vi "Tx_Create FIFO Association - Acyclic Labels - Parameters Channels.vi"(8 "error in (no error)":errorcluster, 11 "Input Channel Data []":T5[](array[typedef]) {"Labels Settings"."Label Timestamp Channel Data Reference" format="%.0x"; "Labels Settings"."Label Disable/Trigger Channel Reference" format="%.0x"; "Labels Settings"."Word"."Param Setting"."Item Refs" format="%.0x"; "Labels Settings"."Word"."Param Setting"."Num Bits" min=1 max=32; "Labels Settings"."Word"."Param Setting"."Start Bit" min=8 max=31; "Labels Settings"."Label" format="%.0o"}) -> (0 "error out":errorcluster, 2 "Raw Values":T1, 3 "Map":T4[](array[typedef]) {"Channel Data Reference" format="%.0x"})   [LabVIEW 2020, in "Ballard Arinc-429 Engine.lvlib"]
doc: "This VI creates a static association between NI-VS FIFO Channel Index and Physical Channel, Label Index, Parameter Index for an Acyclic Tx Label."
uses:
  Ballard Arinc-429 Engine.lvlib
  Shared/Controls and Global/RT HW Channel.ctl
  Shared/Controls and Global/RT Label Settings.ctl
  Shared/Controls and Global/Label.ctl
  Shared/Controls and Global/transferPeriod.ctl
  Shared/Controls and Global/RT Word Settings.ctl
  Shared/Controls and Global/RT Param Setting.ctl
  Shared/Controls and Global/Start Bit.ctl
  Shared/Controls and Global/Number of Bits.ctl
  <vilib>/NI VeriStand/Custom Device API/Block Data Reference.ctl
  <vilib>/NI VeriStand/Custom Device API/Data Reference.ctl
  <vilib>/NI VeriStand/Custom Device API/Custom Device Item Ref.ctl
  Shared/Controls and Global/TransferType.ctl
  RT Controls/RT Tx Association.ctl
  RT Controls/RT Tx Default Raw Value.ctl
  RT Controls/RT Tx Default Raw Value_Association.ctl
  <vilib>/NI VeriStand/Custom Device API/Custom Device API.lvlib
  Shared/Ballard Arinc-429 Shared.lvlib
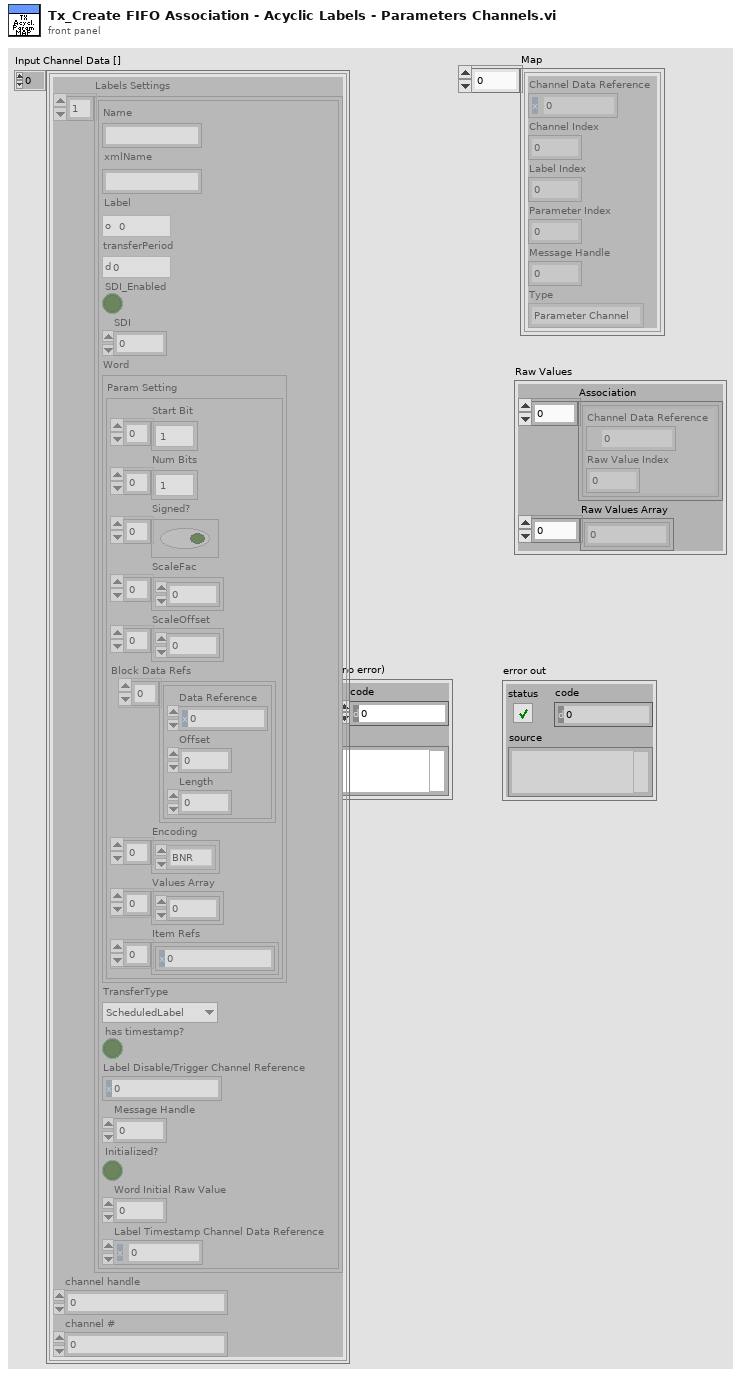
[diagram p1: front panel]
types:
  T1 = typedef "Ballard Arinc-429 Engine.lvlib/RT Tx Default Raw Value.ctl" = cluster{"Association":T2[], "Raw Values Array":u32[]}
  T2 = typedef "Ballard Arinc-429 Engine.lvlib/RT Tx Default Raw Value_Association.ctl" = cluster{"Channel Data Reference":T3, "Raw Value Index":i32}
  T3 = typedef "Custom Device API.lvlib/Data Reference.ctl" = i32
  T4 = typedef "Ballard Arinc-429 Engine.lvlib/RT Tx Association.ctl" = cluster{"Channel Data Reference":T3, "Channel Index":i32, "Label Index":i32, "Parameter Index":i32, "Message Handle":u64, "Type":enum16{"Parameter Channel", "Disable/Trigger Channel"}}
  T5 = typedef "Ballard Arinc-429 Shared.lvlib/RT HW Channel.ctl" = cluster{"Labels Settings":T6[], "channel handle":u64, "channel #":u16}
  T6 = typedef "Ballard Arinc-429 Shared.lvlib/RT Label Settings.ctl" = cluster{"Name":string, "xmlName":string, "Label":T7, "transferPeriod":T8, "SDI_Enabled":bool, "SDI":u8, "Word":T9, "TransferType":T15, "has timestamp?":bool, "Label Disable/Trigger Channel Reference":T14, "Message Handle":u64, "Initialized?":bool, "Word Initial Raw Value":u32, "Label Timestamp Channel Data Reference":T3}
  T7 = typedef "Ballard Arinc-429 Shared.lvlib/Label.ctl" = u8
  T8 = typedef "Ballard Arinc-429 Shared.lvlib/transferPeriod.ctl" = u32
  T9 = typedef "Ballard Arinc-429 Shared.lvlib/RT Word Settings.ctl" = cluster{"Param Setting":T10}
  T10 = typedef "Ballard Arinc-429 Shared.lvlib/RT Param Setting.ctl" = cluster{"Start Bit":T11[], "Num Bits":T12[], "Signed?":bool[], "ScaleFac":dbl[], "ScaleOffset":dbl[], "Block Data Refs":T13[], "Encoding":enum16{"BNR", "BCD", "Discrete"}[], "Values Array":dbl[], "Item Refs":T14[]}
  T11 = typedef "Ballard Arinc-429 Shared.lvlib/Start Bit.ctl" = i32
  T12 = typedef "Ballard Arinc-429 Shared.lvlib/Number of Bits.ctl" = i32
  T13 = typedef "Custom Device API.lvlib/Block Data Reference.ctl" = cluster{"Data Reference":T3, "Offset":u64, "Length":u64}
  T14 = typedef "Custom Device API.lvlib/Custom Device Item Ref.ctl" = u64
  T15 = typedef "Ballard Arinc-429 Shared.lvlib/TransferType.ctl" = enum16{"ScheduledLabel", "Acyclic", "Block", "Strobe"}
  T16 = enum16{"Parameter Channel", "Disable/Trigger Channel"}
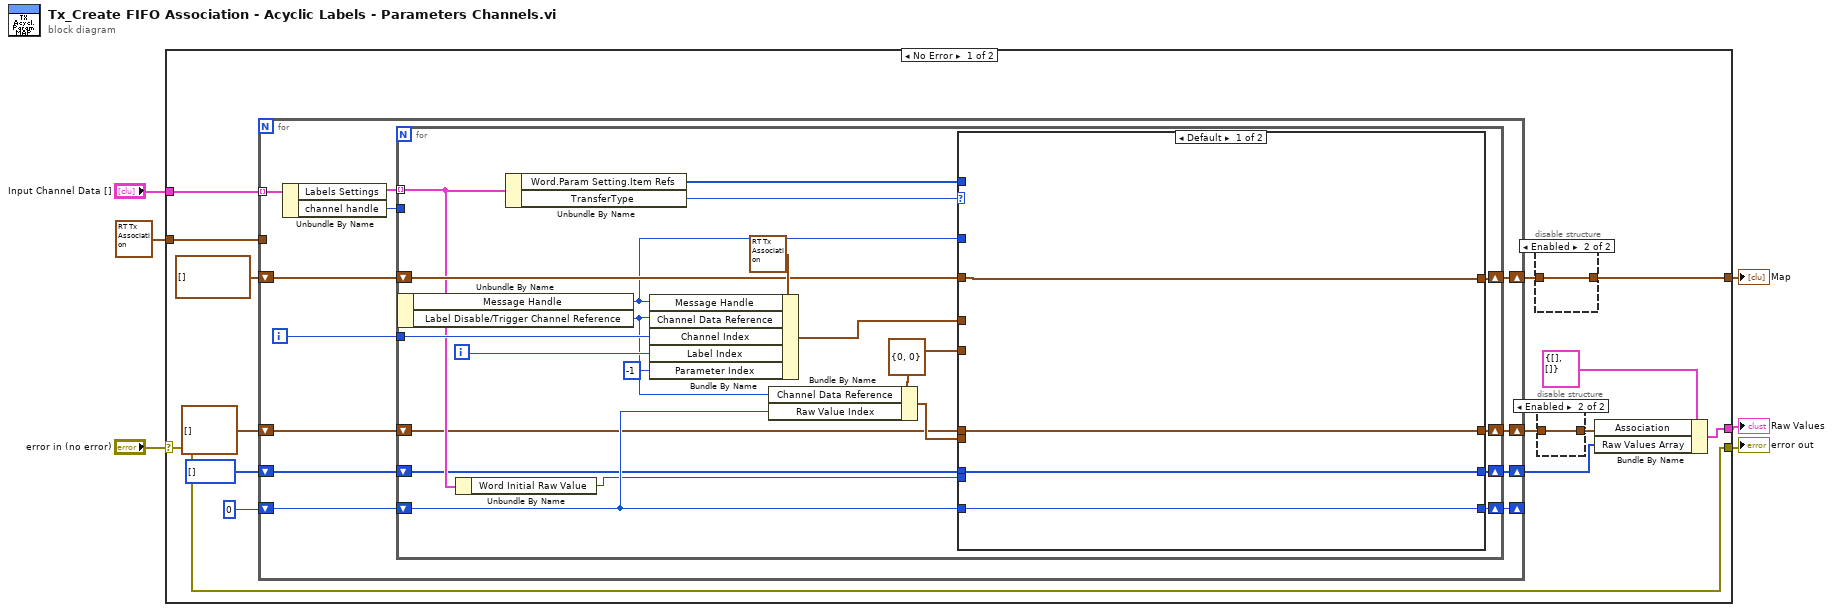
[diagram p0: block diagram]
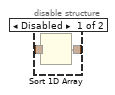
[diagram p2: hidden frame]
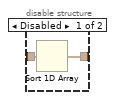
[diagram p3: hidden frame]
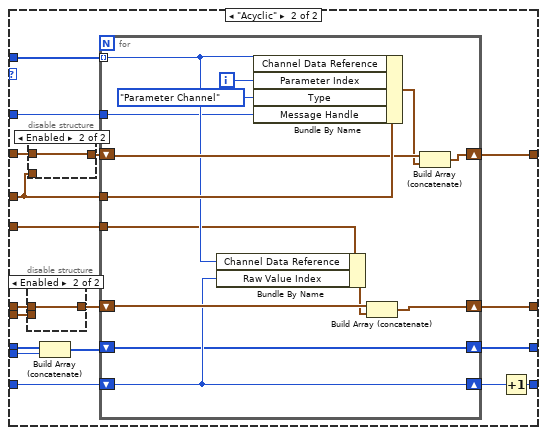
[diagram p4: hidden frame]
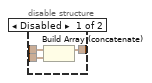
[diagram p5: hidden frame]
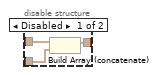
[diagram p6: hidden frame]
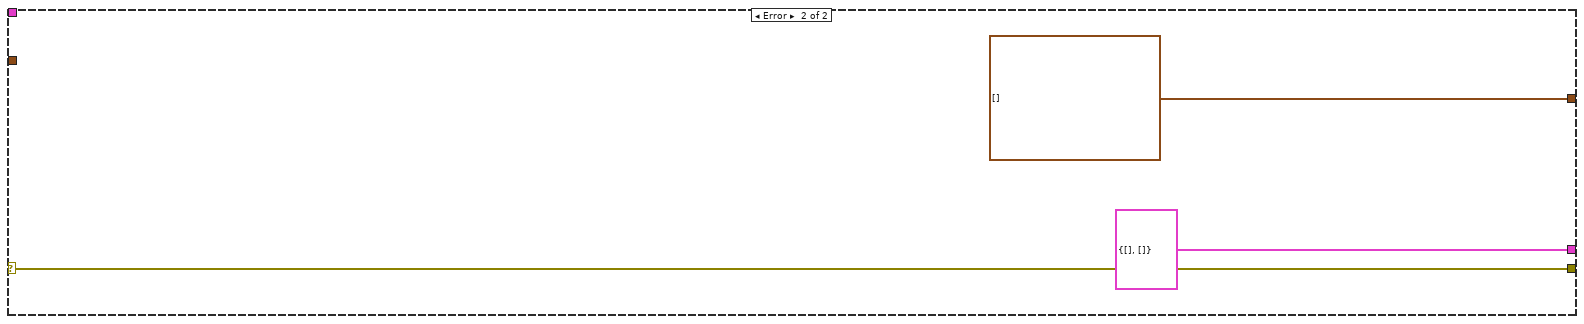
[diagram p7: hidden frame]
diagram:
  n1 = case shown="No Error" "error in (no error)" {
    selector: "error in (no error)" -> [w17 w106]
    tunnel: [w17 w106] -> w5
    tunnel: "Input Channel Data []" -> [w20 _]
    tunnel: T4 {"Channel Data Reference"=0, "Channel Index"=0, "Label Index"=0, "Parameter Index"=0, "Message Handle"=0, "Type"=enum."Parameter Channel"} ("Association") -> [w19 _]
    tunnel: [w16 T4[] []] -> w2
    tunnel: [w12 T1 {"Association"=[], "Raw Values Array"=[]}] -> w1
    frame No Error {
      n2 = for {
        tunnel: w20 -> [w37] mode=indexing
        tunnel: w19 -> [_]
        shift-right: [w34] -> w9
        shift-left: T4[] [] -> [w36]
        shift-right: [w32] -> w8
        shift-left: T2[] [] -> [w33]
        shift-right: [w28] -> w7
        shift-left: u32[] [] -> [w31]
        shift-right: [w29] -> _
        shift-left: 0 -> [w30]
        i -> [w35]
        n3 = Unbundle By Name(w37) -> ("Labels Settings"=w38:T6[], "channel handle"=w27:u64)
        n4 = for {
          tunnel: w38 -> [w51] mode=indexing
          shift-right: [w56] -> w34
          shift-left: w36 -> [w57]
          tunnel: w35 -> [w58]
          shift-right: [w52] -> w32
          shift-left: w33 -> [w45]
          shift-right: [w50] -> w28
          shift-left: w31 -> [w44]
          shift-right: [w49] -> w29
          shift-left: w30 -> [w48]
          tunnel: w27 -> [_]
          i -> [w53]
          w47 = T2 {"Channel Data Reference"=0, "Raw Value Index"=0}
          n5 = Unbundle By Name(w51) -> ("Message Handle"=w41:u64, "Label Disable/Trigger Channel Reference"=w42:T14)
          n6 = Unbundle By Name(w51) -> ("Word Initial Raw Value"=w43:u32)
          n7 = Unbundle By Name(w51) -> ("Word.Param Setting.Item Refs"=w54:T14[], "TransferType"=w40:T15)
          n8 = Bundle By Name(cluster=T4 {"Channel Data Reference"=0, "Channel Index"=0, "Label Index"=0, "Parameter Index"=-1, "Message Handle"=0, "Type"=enum."Disable/Trigger Channel"} ("Association"), "Message Handle"=w41, "Channel Data Reference"=w42, "Channel Index"=w58, "Label Index"=w53, "Parameter Index"=-1) -> (w55:T4)
          n9 = Bundle By Name(cluster=w47, "Channel Data Reference"=w42, "Raw Value Index"=w48) -> (w46:T2)
          n10 = case shown="Default" w40 {
            tunnel: w57 -> [w63 w81]
            tunnel: [w63 w79] -> w56
            tunnel: w55 -> [_ w78]
            tunnel: w54 -> [_ w77]
            tunnel: [w62 w76] -> w52
            tunnel: [w61 w75] -> w50
            tunnel: [w60 w73] -> w49
            tunnel: w48 -> [w60 w72]
            tunnel: w47 -> [_ w71]
            tunnel: w46 -> [_ w70]
            tunnel: w45 -> [w62 w69]
            tunnel: w44 -> [w61 w67]
            tunnel: w43 -> [_ w66]
            tunnel: w41 -> [_ w64]
            frame Default {
            }
            frame "Acyclic" {
              n11 = disable-structure shown="Enabled" {
                disable-tunnel: w70 -> [w84 _]
                disable-tunnel: w69 -> [w83 w85]
                disable-tunnel: [w82 w85] -> w68
                frame Disabled {
                  n12 = Build Array (concatenate)(w83, w84) -> (w82:T2[])
                }
                frame Enabled {
                }
              }
              n13 = disable-structure shown="Enabled" {
                disable-tunnel: w81 -> [w88 w89]
                disable-tunnel: [w87 w89] -> w80
                disable-tunnel: w78 -> [w86 _]
                frame Disabled {
                  n14 = Build Array (concatenate)(w88, w86) -> (w87:T4[])
                }
                frame Enabled {
                }
              }
              n15 = Build Array (concatenate)(w67, w66) -> (w65:u32[])
              n16 = for {
                shift-right: [w100] -> w79
                shift-left: w80 -> [w102]
                tunnel: w78 -> [w103]
                tunnel: w77 -> [w95] mode=indexing
                shift-right: [w97] -> w76
                shift-left: w68 -> [w98]
                shift-right: [w92] -> w75
                shift-left: w65 -> [w92]
                shift-right: [w96] -> w74
                shift-left: w72 -> [w96]
                tunnel: w71 -> [w93]
                tunnel: w64 -> [w91]
                i -> [w99]
                n17 = Bundle By Name(cluster=w93, "Channel Data Reference"=w95, "Raw Value Index"=w96) -> (w94:T2)
                n18 = Bundle By Name(cluster=w103, "Channel Data Reference"=w95, "Parameter Index"=w99, "Type"=T16."Parameter Channel", "Message Handle"=w91) -> (w101:T4)
                n19 = Build Array (concatenate)(w98, w94) -> (w97:T2[])
                n20 = Build Array (concatenate)(w102, w101) -> (w100:T4[])
              }
              n21 = Increment(x=w74) -> (x+1=w73:i32)
            }
          }
        }
      }
      n22 = disable-structure shown="Enabled" {
        disable-tunnel: w9 -> [w25 w26]
        disable-tunnel: [w24 w26] -> w16
        frame Disabled {
          n23 = Sort 1D Array(array=w25) -> (sorted array=w24:T4[])
        }
        frame Enabled {
        }
      }
      n24 = disable-structure shown="Enabled" {
        disable-tunnel: w8 -> [w22 w23]
        disable-tunnel: [w21 w23] -> w13
        frame Disabled {
          n25 = Sort 1D Array(array=w22) -> (sorted array=w21:T2[])
        }
        frame Enabled {
        }
      }
      n26 = Bundle By Name(cluster=T1 {"Association"=[], "Raw Values Array"=[]} ("Raw Values"), "Association"=w13, "Raw Values Array"=w7) -> (w12:T1)
    }
    frame Error {
    }
  }
  "error out" <- w5
  "Map" <- w2
  "Raw Values" <- w1
